vi "ROI group-Highlight group in ctrl.vi"(7 "Value signalling?":bool, 8 "error in (no error)":errorcluster, 11 "Index of group to update":i16) -> (0 "error out":errorcluster)   [LabVIEW 2020]
uses:
  Global variables/gl_Functional Imaging-Global variables.vi
  ROI grouping window/Globals/gl_ROI grp window globals.vi
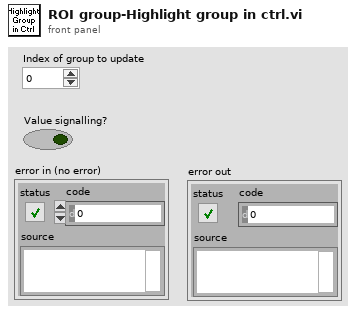
[diagram p1: front panel]
types:
  T1 = typedef "Functional Imging UI Refs.ctl" = cluster{"Menu ref":refnum<k9>, "Image control":refnum<vi>, "VI ref":refnum<vi>, "XGrapher":refnum<vi>, "Smoothing":refnum<vi>, "POI Averaging":refnum<vi>, "Normalize":refnum<vi>, "POI data points in each trial":refnum<vi>, "Channel":refnum<vi>, "Experiment data folder path":refnum<vi>, "[ROI vis]":refnum<vi>, "[Groups] visbl":T2, "Group Name":refnum<vi>, "POI index":refnum<vi>, "Trial No.":refnum<vi>, "Intensity Zoom":refnum<vi>, "Trial Cursor Enabled":refnum<vi>, "Number of Trials (ind 1)":refnum<vi>, "Number of Trials (ind 2)":refnum<vi>, "MiniScans Available":refnum<vi>, "POI Available":refnum<vi>, "Defer graph updates":refnum<vi>, "Waveform selector":refnum<vi>, "#of selected POI":refnum<vi>, "#of selected MiniScans":refnum<vi>, "#of selected groups":refnum<vi>, "Max Z-Projection":refnum<vi>, "Z-Plane Selector":refnum<vi>, "Index of miniscan point to visualise":refnum<vi>, "ROI vis. mode":refnum<vi>, "Total # of points":refnum<vi>, "Index of group clicked on":refnum<vi>, "Pane 1":refnum<vi>, "Pane 2":refnum<vi>, "Pane 3":refnum<vi>, "Pane 4":refnum<vi>, "Pane 5":refnum<vi>, "Pane 6":refnum<vi>, "Deselect all ROI":refnum<vi>, "Deselect all groups":refnum<vi>}
  T2 = typedef "Groups array referecne.ctl" = refnum<vi>
  T3 = typedef "Group sel cluster.ctl" = cluster{"Group number":string, "Group Name":string, "Visibility":bool, "Highlight":bool}
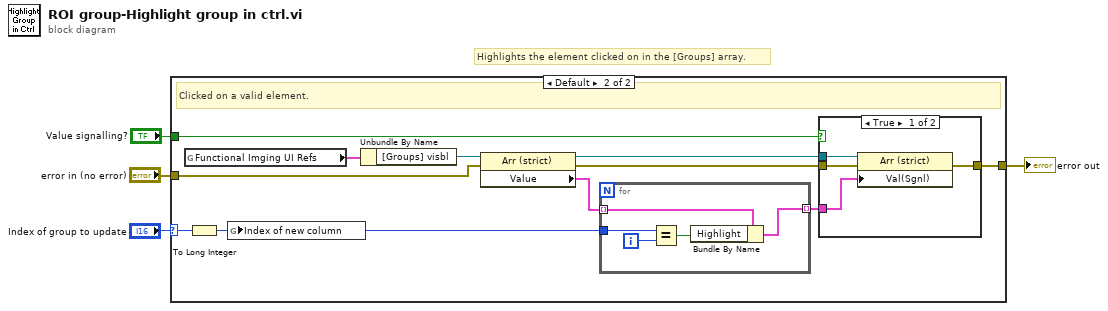
[diagram p0: block diagram]
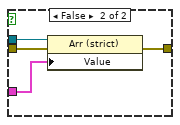
[diagram p3: hidden frame]
diagram:
  # "Highlights the element clicked on in the [Groups] array."
  n1 = case shown="Default" "Index of group to update" {
    selector: "Index of group to update" -> [_ w7]
    tunnel: "error in (no error)" -> [w5 w14]
    tunnel: [w5 w9] -> w3
    tunnel: "Value signalling?" -> [_ w8]
    frame -1 {
    }
    frame Default {
      # "Clicked on a valid element."
      n2 = global read "gl_Functional Imaging-Global variables.vi" "Functional Imging UI Refs"() -> (w12:T1)
      n3 = To Long Integer(number=w7) -> (32bit integer=w6:i32)
      n4 = global write "gl_ROI grp window globals.vi" "Index of new column"(w6) -> ()
      n5 = Unbundle By Name(w12) -> ("[Groups] visbl"=w15:T2)
      n6 = property on="Property Node" class="Arr (strict)"(reference=w15, error in=w14) -> (reference out=w16:T2, error out=w13:errorcluster, "Value"=w11:T3[])
      n7 = for {
        tunnel: w11 -> [w29] mode=indexing
        tunnel: [w28] -> w10 mode=indexing
        tunnel: w6 -> [w26]
        i -> [w27]
        n8 = Equal?(x=w26, y=w27) -> (x = y?=w25:bool)
        n9 = Bundle By Name(cluster=w29, "Highlight"=w25) -> (w28:T3)
      }
      n10 = case shown="True" w8 {
        tunnel: w16 -> [w20 w24]
        tunnel: w13 -> [w19 w23]
        tunnel: w10 -> [w18 w22]
        tunnel: [w17 w21] -> w9
        frame True {
          n11 = property on="Property Node" class="Arr (strict)"(reference=w20, error in=w19, "Val(Sgnl)"=w18) -> (error out=w17:errorcluster)  [unwired: 1 out]
        }
        frame False {
          n12 = property on="Property Node" class="Arr (strict)"(reference=w24, error in=w23, "Value"=w22) -> (error out=w21:errorcluster)  [unwired: 1 out]
        }
      }
    }
  }
  "error out" <- w3
